vi "GetPkToAvPowerN1911a.vi"(2 "error in (no error)":errorcluster) -> (0 "Error out":errorcluster, 1 "Power returned (dBm)":dbl format="%#.10f")   [LabVIEW 2009]
doc: "Reads the power from the N1911A power meter."
panel:
  # "Get Peak-to-aver power from N1911A insure that calc3:feed1 is set to PTAV)"
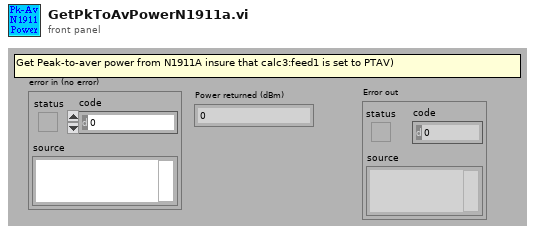
[diagram p1: front panel]
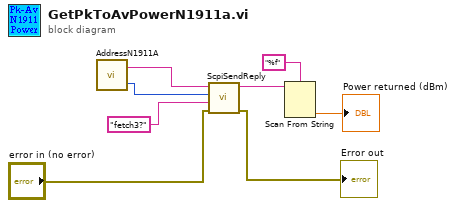
[diagram p0: block diagram]
diagram:
  n1 = call "AddressN1911A.vi"() -> ("Port"=w2:i32, "IP address"=w1:string)  [unwired: 2 in]
  n2 = call "ScpiSendReply.vi"("error in (no error)"="error in (no error)", "Command"="fetch3?" ("format string"), "TCP port"=w2, "IP Address"=w1) -> ("Error out"=→"Error out":errorcluster, "Reply"=w6:string)  [unwired: 5 in]
  n3 = Scan From String(format string="%f", input string=w6) -> (output 1=→"Power returned (dBm)":dbl)  [unwired: 3 in, 3 out]
